vi "Maps-Set Zoom.vi"(0 "Google Maps Resource Out in":T1, 7 "Zoom":i32, 11 "error in (no error)":errorcluster) -> (4 "Google Maps Resource Out out":T1, 15 "error out":errorcluster)   [LabVIEW 2020]
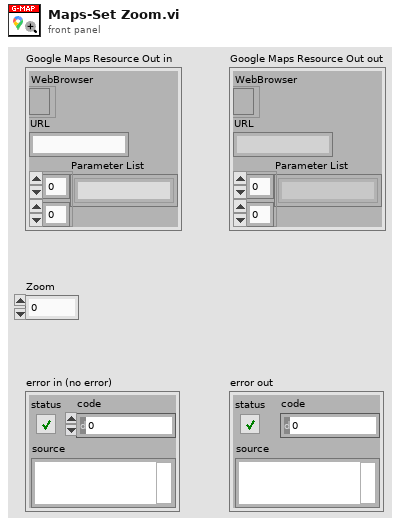
[diagram p1: front panel]
types:
  T1 = cluster{"WebBrowser":refnum<k7>, "URL":string, "Parameter List":string[][]}
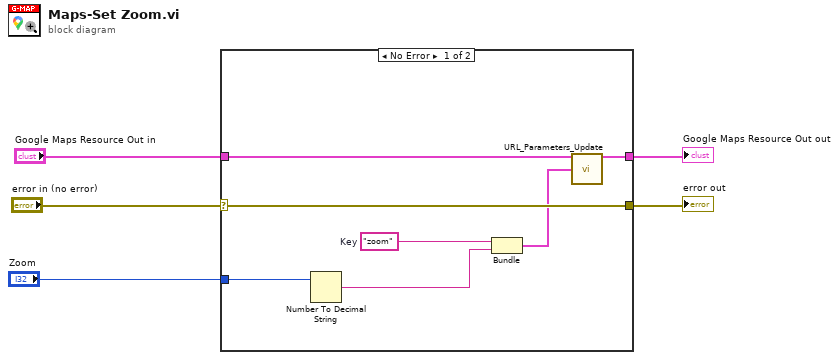
[diagram p0: block diagram]
diagram:
  n1 = case shown="No Error" "error in (no error)" {
    selector: "error in (no error)" -> [w12 w13]
    tunnel: "Google Maps Resource Out in" -> [w10 w14]
    tunnel: [w8 w14] -> w2
    tunnel: [w12 w13] -> w4
    tunnel: "Zoom" -> [w7 _]
    frame No Error {
      w11 = "zoom"  # Key
      n2 = Number To Decimal String(number=w7) -> (decimal integer string=w6:string)  [unwired: 1 in]
      n3 = Bundle("Key"=w11, w6) -> (w9:cluster{"Key":string, string})  [unwired: 1 in]
      n4 = call "URL_Parameters_Update.vi"("Google Maps Resource In"=w10, "URL Parameter"=w9) -> ("Google Maps Resource Out"=w8:T1)  [unwired: 13 in]
    }
    frame Error {
    }
  }
  "error out" <- w4
  "Google Maps Resource Out out" <- w2
